vi "demo.vi"() -> ()   [LabVIEW 2011]
panel:
  in  "基路径":path
  in  "xml_info":T1={"FileVersion"="DevelopmentSystem", "FileName"="DevelopmentSystem", "test time"=["2016/11/14 11:59:03"], "original Path"=path "D:/高频房软件/2. HPTS_VNA_Rev2.7.1.3-1107最新源码/Demo_data", "show_TDD11"=[], "show_TDD22"=[], "show_impspec"=[], "usedSN"="", "diffspec"={"limit Spec"=[], "Diff Test Item Name"=[], "Spec _Col"=[]}, "secondresult"=[], "show_Terminal Point"=[], "show_Cable Point"=[], "customerPN"="", "auto get refer point"=FALSE, "width1"=0, "width2"=0}
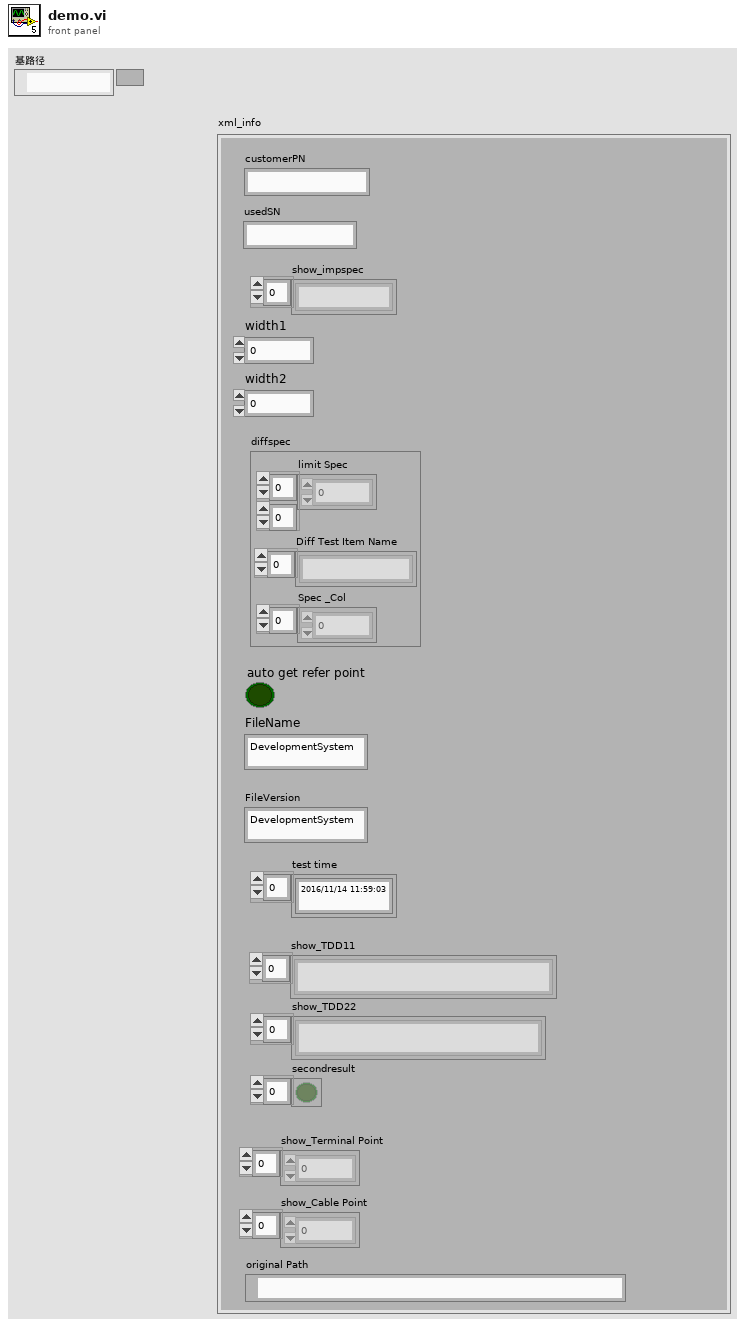
[diagram p1: front panel]
types:
  T1 = cluster{"FileVersion":string, "FileName":string, "test time":string[], "original Path":path, "show_TDD11":string[], "show_TDD22":string[], "show_impspec":string[], "usedSN":string, "diffspec":cluster{"limit Spec":dbl[][], "Diff Test Item Name":string[], "Spec _Col":i32[]}, "secondresult":bool[], "show_Terminal Point":dbl[], "show_Cable Point":dbl[], "customerPN":string, "auto get refer point":bool, "width1":i32, "width2":i32}
  T2 = enum16{"MINI SAS HD 4X", "MINI SAS 4X", "SFP28", "QSFP28"}
  T3 = cluster{"limit Spec":dbl[][], "Diff Test Item Name":string[], "Spec _Col":i32[]}
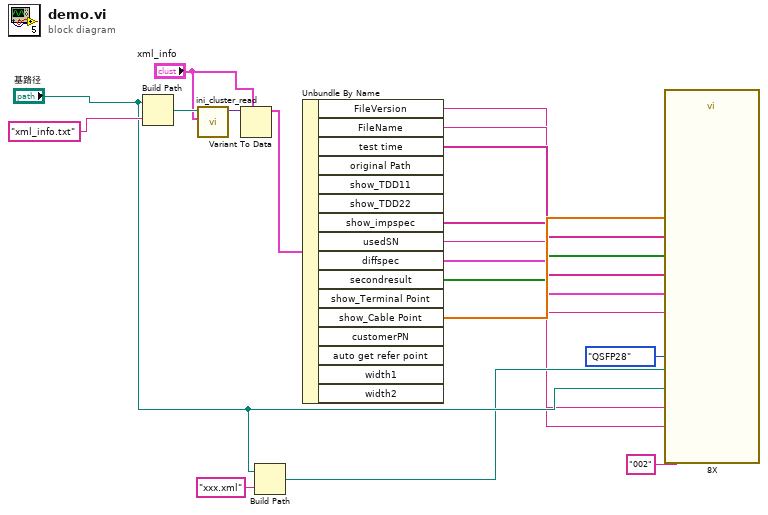
[diagram p0: block diagram]
diagram:
  n1 = Build Path(base path="基路径", name or relative path="xml_info.txt" ("名称或相对路径")) -> (appended path=w18:path)
  n2 = call "ini_cluster_read.vi"("INI Fomatted Cluster Type"="xml_info", "configuration file path"=w18) -> ("ini cluster out"=w17:variant)  [unwired: 8 in, 1 out]
  n3 = Variant To Data(type="xml_info", Variant=w17) -> (data=w14:T1)  [unwired: 1 in, 1 out]
  n4 = Build Path(base path="基路径", name or relative path="xxx.xml" ("名称或相对路径")) -> (appended path=w5:path)
  n5 = Unbundle By Name(w14) -> ("FileVersion"=w2:string, "FileName"=w3:string, "test time"=w12:string[], "show_impspec"=w11:string[], "usedSN"=w9:string, "diffspec"=w10:T3, "secondresult"=w4:bool[], "show_Cable Point"=w13:dbl[])  [unwired: 8 out]
  n6 = call "8X.vi"("xml path"=T2."QSFP28" ("type"), "type"=w10, 2:"002" ("input_str_CustomerPN"), 3:w9, 4:"基路径", "txtPath"=w11, 6:w12, "singleItemInfo"=w13, 10:w5, "TDD"=w3, 12:w4, 13:w2) -> ()  [unwired: 4 in]
